vi "EventsDemo.vi"() -> ()   [LabVIEW 2011]
doc: "Use this template to build a user interface event handler design pattern. Use this pattern for dialog boxes and other user interfaces. You also can create and execute user-defined events that the VI can handle the same way as user interface events."
panel:
  out "Blink":bool
  in  "Blink Rate (ms)":i32
  in  "Value In":dbl(slide) scale=0.0..10.0
  out "Last Button":cluster{"1":bool, "2":bool, "3":bool}
  out "2 x Value":dbl
  in  "Button 3":bool
  in  "Button 2":bool
  in  "Button 1":bool
  in  "stop":bool
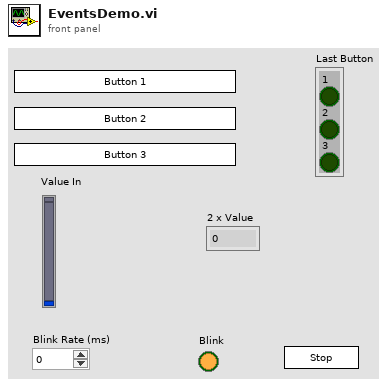
[diagram p1: front panel]
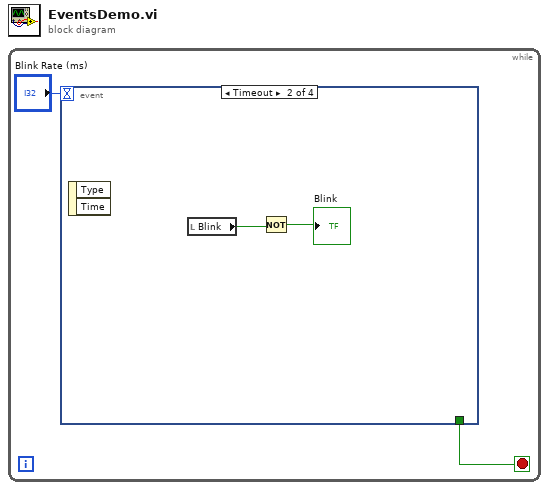
[diagram p0: block diagram]
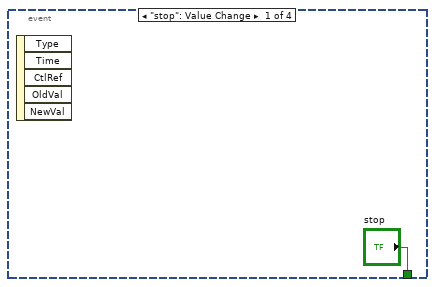
[diagram p2: hidden frame]
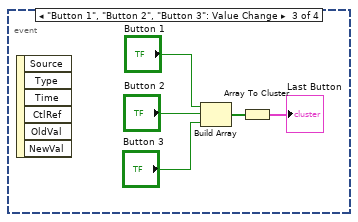
[diagram p3: hidden frame]
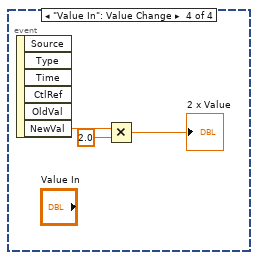
[diagram p4: hidden frame]
diagram:
  n1 = while {
    stop <- w2 stop-if-true
    n2 = event shown="[1] Timeout" {
      selector: _ -> [_ _ _ _]
      dyn-events: _ -> [_ _ _ _]
      timeout: "Blink Rate (ms)" -> [_ _ _ _]
      tunnel: ["stop" _ _ _] -> w2
      event "stop": Value Change {
        n3 = event-data() -> ()  [unwired: 1 in, 5 out]
      }
      event Timeout {
        n4 = event-data() -> ()  [unwired: 1 in, 2 out]
        n5 = local read "Blink"() -> (w5:bool)
        n6 = Not(x=w5) -> (.not. x?=→"Blink":bool)
      }
      event "Button 1", "Button 2", "Button 3": Value Change {
        n7 = event-data() -> ()  [unwired: 1 in, 6 out]
        n8 = Build Array("Button 1", "Button 2", "Button 3") -> (w7:bool[])
        n9 = Array To Cluster(array=w7) -> (cluster=→"Last Button":cluster{"[0]":bool, "[1]":bool, "[2]":bool})
      }
      event "Value In": Value Change {
        n10 = event-data() -> ("NewVal"=w13:dbl)  [unwired: 1 in, 5 out]
        n11 = Multiply(x=w13, y=2.0) -> (x*y=→"2 x Value":dbl)
      }
    }
  }
